vi "Write frequency.vi"(8 "error in (no error)":errorcluster, 10 "frequency":dbl, 11 "Signal Waveform in":refnum<class "Signal Waveform.lvclass">) -> (0 "error out":errorcluster, 3 "Signal Waveform out":refnum<class "Signal Waveform.lvclass">)   [LabVIEW 2020, in "Signal Waveform.lvclass"]
uses:
  Signal Waveform.lvclass
  Signal Waveform.lvclass/Signal Waveform.ctl
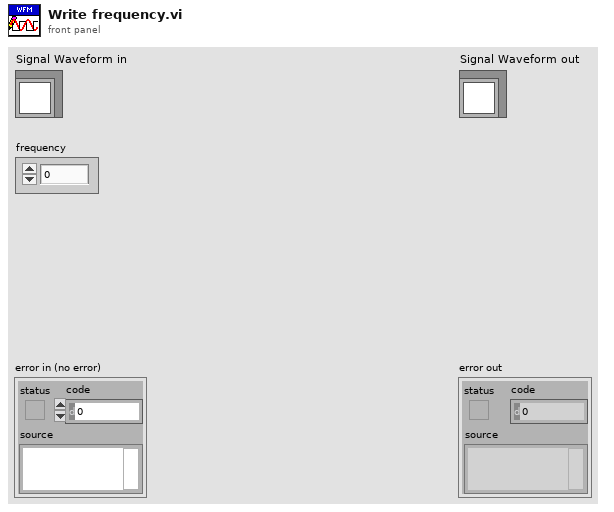
[diagram p1: front panel]
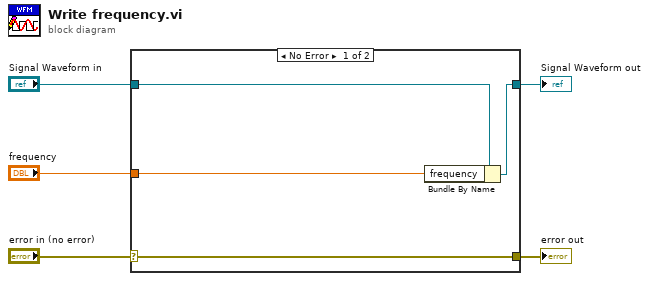
[diagram p0: block diagram]
diagram:
  n1 = case shown="No Error" "error in (no error)" {
    selector: "error in (no error)" -> [w9 w10]
    tunnel: [w9 w10] -> w4
    tunnel: [w7 w11] -> w2
    tunnel: "Signal Waveform in" -> [w8 w11]
    tunnel: "frequency" -> [w6 _]
    frame No Error {
      n2 = Bundle By Name(cluster=w8, "frequency"=w6) -> (w7:refnum<class "Signal Waveform.lvclass">)
    }
    frame Error {
    }
  }
  "error out" <- w4
  "Signal Waveform out" <- w2
